vi "SolicitarLimites.vi"(8 "error in (no error)":errorcluster, 10 "Limites":T1, 11 "Limites Contador in":refnum<class "Limites Contador.lvclass">) -> (0 "error out":errorcluster, 3 "Limites Contador out":refnum<class "Limites Contador.lvclass">)   [LabVIEW 2020, in "Limites Contador.lvlib" / "Limites Contador.lvclass"]
uses:
  Limites Contador.lvclass
  Limites Contador.lvclass/Limites Contador.ctl
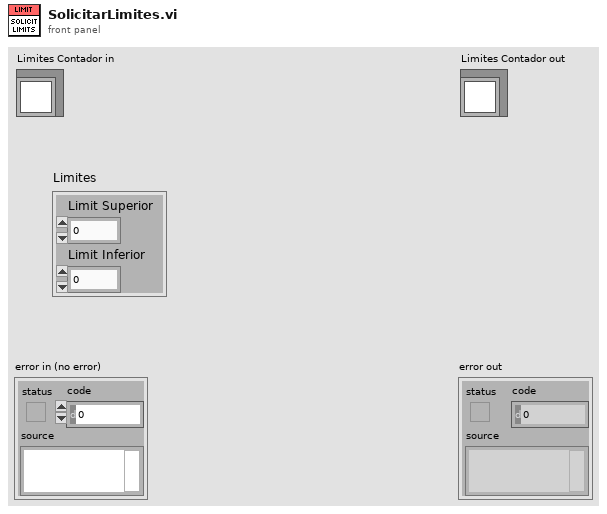
[diagram p1: front panel]
types:
  T1 = cluster{"Limit Superior":dbl, "Limit Inferior":dbl}
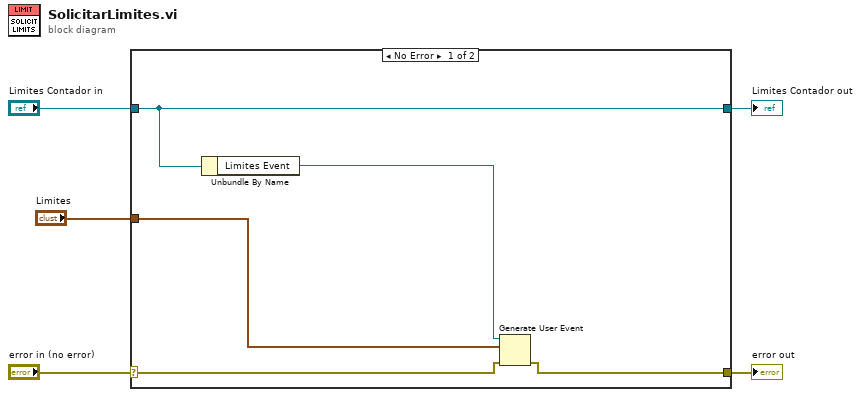
[diagram p0: block diagram]
diagram:
  n1 = case shown="No Error" "error in (no error)" {
    selector: "error in (no error)" -> [w8 w12]
    tunnel: [w9 w12] -> w4
    tunnel: [w10 w11] -> w2
    tunnel: "Limites Contador in" -> [w10 w11]
    tunnel: "Limites" -> [w6 _]
    frame No Error {
      n2 = Unbundle By Name(w10) -> ("Limites Event"=w7:refnum<user-event>)
      n3 = Generate User Event(user event=w7, event data cluster=w6, error in=w8) -> (error out=w9:errorcluster)  [unwired: 1 in, 1 out]
    }
    frame Error {
    }
  }
  "error out" <- w4
  "Limites Contador out" <- w2
